vi "Read Sender.vi"(11 "Destroy Msg in":refnum<class "Destroy Msg.lvclass">) -> (2 "Sender":refnum<class "Sender.lvclass">)   [LabVIEW 2025, in "jettl.lvlib" / "Destroy Msg.lvlib" / "Destroy Msg.lvclass"]
uses:
  Destroy Msg.lvclass
  Sender/Sender/Sender.lvclass
  Destroy Msg.lvclass/Destroy Msg.ctl
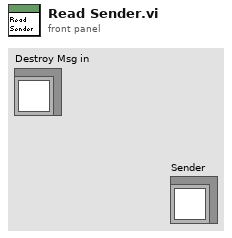
[diagram p1: front panel]
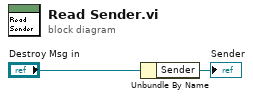
[diagram p0: block diagram]
diagram:
  n1 = Unbundle By Name("Destroy Msg in") -> ("Sender"=→"Sender":refnum<class "Sender.lvclass">)
